vi "advancedOpenNoClose.vi"() -> ()   [LabVIEW 2026]
panel:
  out "10 second countdown":i32
  out "appended path":path
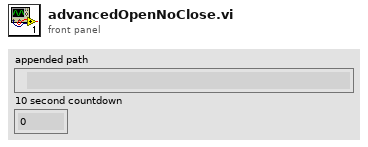
[diagram p1: front panel]
types:
  T1 = enum16{"open", "open or create", "create or replace", "create", "open (read-only)"}
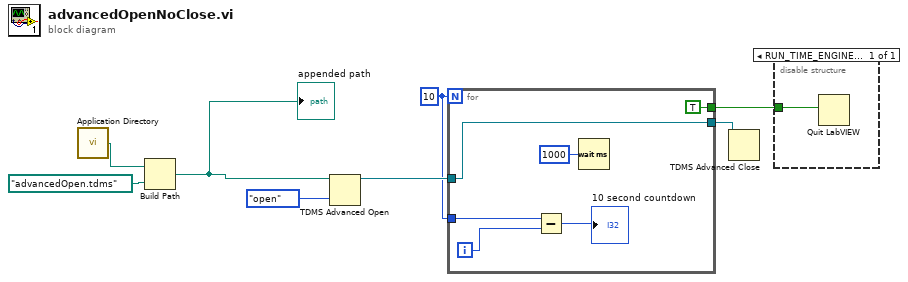
[diagram p0: block diagram]
diagram:
  w3 = 10
  n1 = call <vilib>:"Application Directory.vi"() -> ("Application Directory"=w8:path)
  n2 = Build Path(base path=w8, name or relative path=path "advancedOpen.tdms") -> (appended path=w5:path)
  "appended path" <- w5
  n3 = TDMS Advanced Open(10:T1."open" ("operation (0:open)"), 11:w5) -> (3:w4:refnum<k34>)  [unwired: 3 in, 2 out]
  n4 = for {
    N: w3 -> [_]
    tunnel: w4 -> [w9]
    tunnel: w3 -> [w11]
    tunnel: [TRUE ("quit? (T)")] -> w2
    tunnel: [w9] -> w1
    i -> [w12]
    n5 = Subtract(x=w11, y=w12) -> (x-y=→"10 second countdown":i32)
    n6 = Wait (ms)(milliseconds to wait=u32 1000) -> ()  [unwired: 1 out]
  }
  n7 = TDMS Advanced Close(11:w1) -> ()  [unwired: 3 in, 2 out]
  n8 = disable-structure shown="RUN_TIME_ENGINE==True, Default" {
    disable-tunnel: w2 -> [w15]
    frame condition #0 (active) {
      n9 = Quit LabVIEW(quit? (T)=w15) -> ()
    }
  }
